vi "test Basic Resolution.vi"(8 "error in (no error)":errorcluster, 11 "TestCase in":refnum<class "Result Tests.lvclass">) -> (0 "error out":errorcluster, 3 "TestCase out":refnum<class "Result Tests.lvclass">)   [LabVIEW 2017, in "Result Tests.lvclass"]
uses:
  Result Tests.lvclass
  <vilib>/addons/_JKI Toolkits/VI Tester/TestCase.llb/TestCase.lvclass
  Futures/Result/Result.lvclass
  C:/Program Files (x86)/National Instruments/LabVIEW 2017/vi.lib/addons/_JKI Toolkits/VI Tester/TestCase.llb/TestCase.lvclass
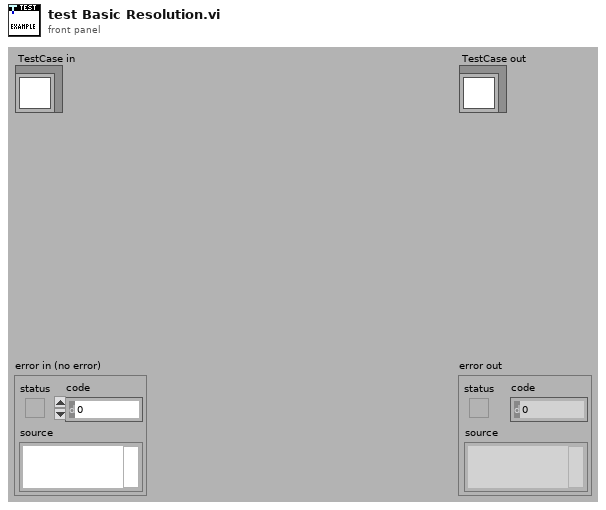
[diagram p1: front panel]
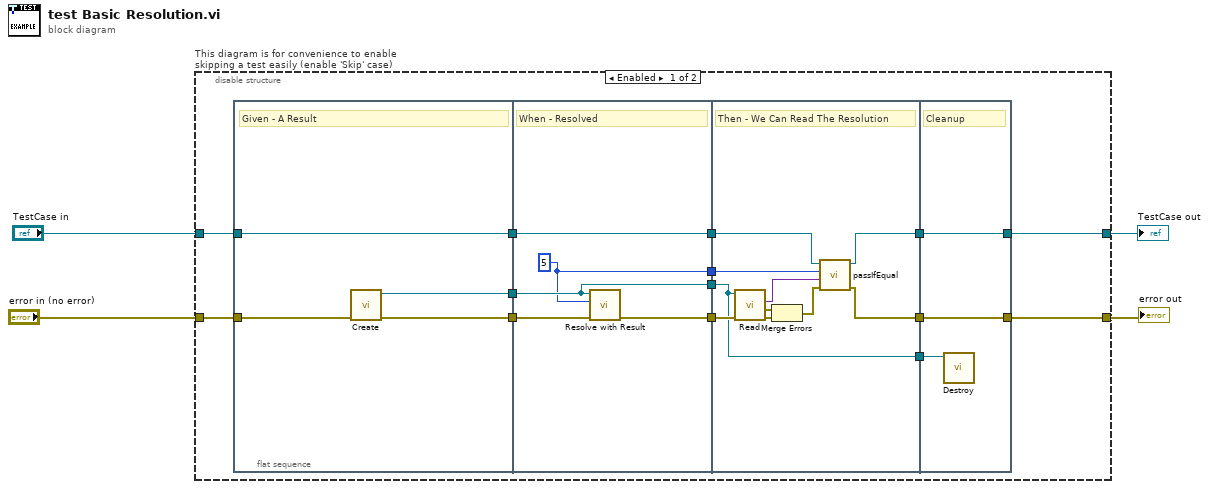
[diagram p0: block diagram]
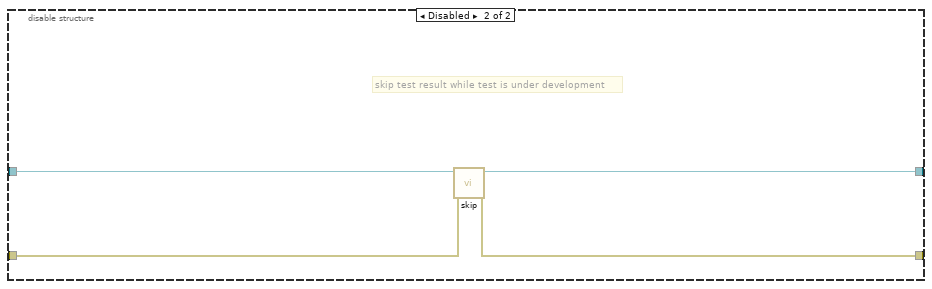
[diagram p2: hidden frame]
diagram:
  n1 = disable-structure "This diagram is for convenience to enable skipping a test easily (enable 'Skip' case)" shown="Enabled" {
    disable-tunnel: "TestCase in" -> [w12 w44]
    disable-tunnel: [w10 w42] -> w1
    disable-tunnel: [w9 w43] -> w3
    disable-tunnel: "error in (no error)" -> [w11 w41]
    frame Enabled {
      n2 = flat-sequence {
        tunnel: w11 -> [w21]
        tunnel: w12 -> [w22]
        tunnel: [w22] -> w18
        tunnel: [w20] -> w17
        tunnel: [w19] -> w8
        tunnel: [w27] -> w16
        tunnel: [w25] -> w15
        tunnel: w18 -> [w27]
        tunnel: w17 -> [w26]
        tunnel: w8 -> [w24]
        tunnel: [w24] -> w7
        tunnel: [w23] -> w6
        tunnel: [w36] -> w14
        tunnel: [w35] -> w13
        tunnel: w16 -> [w37]
        tunnel: w15 -> [w34]
        tunnel: w7 -> [w28]
        tunnel: w6 -> [w29]
        tunnel: [w28] -> w5
        tunnel: [w39] -> w9
        tunnel: [w40] -> w10
        tunnel: w14 -> [w40]
        tunnel: w13 -> [w39]
        tunnel: w5 -> [w38]
        frame #0 {
          # "Given - A Result"
          n3 = call "Create.vi"("error in (no error)"=w21) -> ("error out"=w20:errorcluster, "Result out"=w19:refnum<class "Result.lvclass">)  [unwired: 9 in]
        }
        frame #1 {
          w23 = 5
          # "When - Resolved"
          n4 = call "Resolve with Result.vi"("error in (no error)"=w26, "Result"=w23, "Result in"=w24) -> ("error out"=w25:errorcluster)  [unwired: 8 in]
        }
        frame #2 {
          # "Then - We Can Read The Resolution"
          n5 = call "Read.vi"("error in (no error)"=w34, "Result in"=w28) -> ("error out"=w33:errorcluster, "result error"=w31:errorcluster, "Result value"=w30:variant)  [unwired: 5 in, 2 out]
          n6 = Merge Errors(w31, w33) -> (w32:errorcluster)
          n7 = call-dynamic "passIfEqual.vi"("error in (no error)"=w32, "y"=w30, "x"=w29, "TestCase in"=w37) -> ("error out"=w35:errorcluster, "TestCase out"=w36:refnum<class "Result Tests.lvclass">)  [unwired: 6 in]
        }
        frame #3 {
          # "Cleanup"
          n8 = call "Destroy.vi"("Result in"=w38) -> ()  [unwired: 9 in, 2 out]
        }
      }
    }
    frame Disabled {
      # "skip test result while test is under development"
      n9 = call <vilib>:"skip.vi"("error in (no error)"=w41, "TestCase in"=w44) -> ("error out"=w43:errorcluster, "TestCase out"=w42:refnum<class "Result Tests.lvclass">)  [unwired: 8 in]
    }
  }
  "error out" <- w3
  "TestCase out" <- w1
